vi "Execute.vi"(8 "error in":errorcluster, 11 "Toggle Speaker in":refnum<class "Toggle Speaker.lvclass">) -> (0 "error out":errorcluster, 1 "Next Step?":bool, 2 "MSG":string, 3 "Toggle Speaker out":refnum<class "Toggle Speaker.lvclass">)   [LabVIEW 2014, in "Toggle Speaker.lvclass"]
uses:
  Toggle Speaker.lvclass
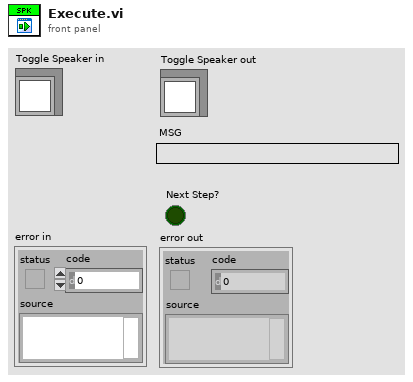
[diagram p1: front panel]
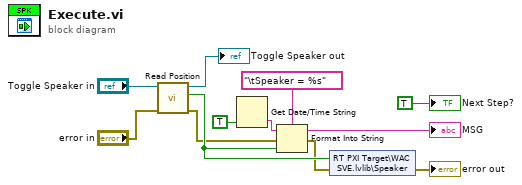
[diagram p0: block diagram]
diagram:
  n1 = call-dynamic "Read Position.vi"("error in"="error in", "Switch Step in"="Toggle Speaker in") -> ("error out"=w2:errorcluster, "Position"=w6:bool, "Switch Step out"=→"Toggle Speaker out":refnum<class "Toggle Speaker.lvclass">)  [unwired: 7 in]
  n2 = Get Date/Time String(want seconds? (F)=TRUE) -> (time string=w5:string)  [unwired: 2 in, 1 out]
  n3 = Format Into String(format string="\tSpeaker = %s", initial string=w5, error in=w2, w6) -> (resulting string=→"MSG":string, error out=w3:errorcluster)
  n4 = shared-variable "RT PXI Target\\WAC SVE.lvlib\\Speaker"(w6, error in=w3) -> (error out=→"error out":errorcluster)
  "Next Step?" <- TRUE ("Next Step?")
